vi "RNG Uniform_DBL.vi"(8 "error in (no error)":errorcluster, 9 "B":dbl, 10 "A":dbl, 11 "RNG in":refnum<class "RNG.lvclass">) -> (0 "error out":errorcluster, 2 "RandomNumber":dbl, 3 "RNG out":refnum<class "RNG.lvclass">)   [LabVIEW 2020, in "OpenLvVision_OpenCv.lvlib" / "RNG.lvclass"]
doc: "Returns uniformly distributed integer random number from [a,b) range"
uses:
  RNG.lvclass
  _LvHelpers/EdvrObject/EdvrObject.lvclass
  OpenLvVision_OpenCv.lvlib
  Dlls/OlvOpenCvWrapper.dll
  C:/Users/lukas/Downloads/OpenLvVision_OpenCv/SourceCode/LabView/OpenLvVision_OpenCv/_LvHelpers/EdvrObject/EdvrObject.lvclass
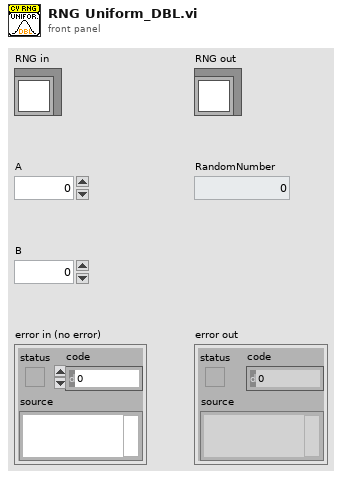
[diagram p1: front panel]
types:
  T1 = typedef "OpenLvVision_OpenCv.lvlib/EdvrObject.lvclass/Edvr.ctl" = refnum<data-value>
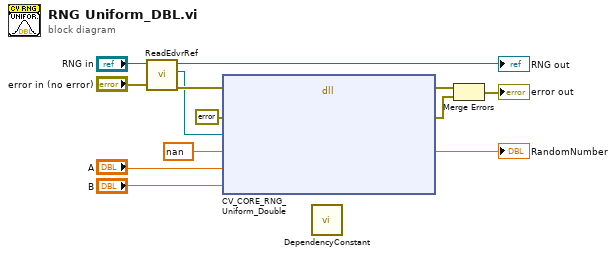
[diagram p0: block diagram]
diagram:
  n1 = call "ReadEdvrRef.vi"("error in (no error)"="error in (no error)", "EdvrObject in"="RNG in") -> ("error out"=w12:errorcluster, "Edvr"=w11:T1, "EdvrObject out"=→"RNG out":refnum<class "RNG.lvclass">)  [unwired: 7 in]
  n2 = dll-call lib="C:/Users/lukas/Downloads/OpenLvVision_OpenCv/SourceCode/LabView/OpenLvVision_OpenCv/Dlls/OlvOpenCvWrapper.dll" fn="CV_CORE_RNG_Uniform_Double"(error in=w12, "Error"=errorcluster {"status"=FALSE, "code"=0, "source"=""} ("error out"), "edvrRef"=w11, "number"=nan, "A"="A", "B"="B") -> (error out=w10:errorcluster, "Error"=w1:errorcluster, "number"=→"RandomNumber":dbl)  [unwired: 6 in, 1 out]
  n3 = call "DependencyConstant.vi"() -> ()  [unwired: 12 in]
  n4 = Merge Errors(w10, w1) -> (→"error out":errorcluster)
